vi "Get SMO Public API.vi"(8 "error in (no error)":errorcluster, 11 "Example Instrument in":refnum<class "Instrument.Element2.lvclass">) -> (0 "error out":errorcluster, 2 "Commands":string[](array[string]), 3 "Example Instrument out":refnum<class "Instrument.Element2.lvclass">)   [LabVIEW 2019, in "Instrument.Element2.lvclass"]
uses:
  Instrument.Element2.lvclass
  Typedefs/Instrument.Element2.Commands--Enum.ctl
  <userlib>/LevyLab/Instrument Framework/Instrument Types/VSource/Instrument.VSource.lvclass
  <userlib>/LevyLab/Instrument Framework/SMOs/Instrument/Instrument.lvclass
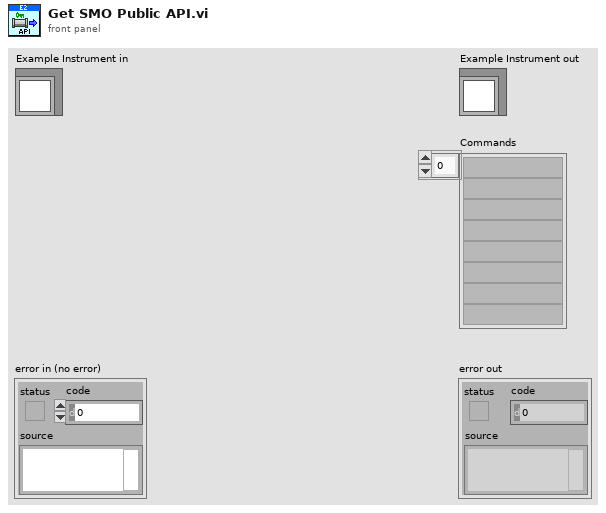
[diagram p1: front panel]
types:
  T1 = typedef "Instrument.Element2.lvclass/Instrument.Element2.Commands--Enum.ctl" = enum16{"command0", "command1", "command2"}
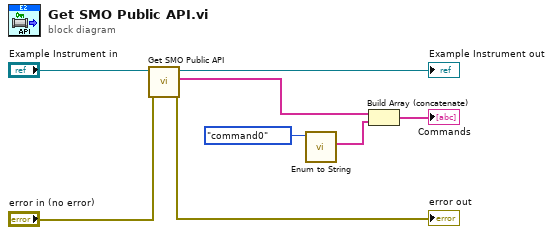
[diagram p0: block diagram]
diagram:
  n1 = call-parent "Get SMO Public API.vi"("error in (no error)"="error in (no error)", "Instrument in"="Example Instrument in") -> ("error out"=→"error out":errorcluster, "Commands"=w8:string[], "Instrument out"=→"Example Instrument out":refnum<class "Instrument.Element2.lvclass">)  [unwired: 7 in]
  n2 = call <userlib>:"Enum to String.vi"("Command"=Instrument.Element2.Commands--Enum."command0" ("Commands")) -> ("Commands []"=w3:string[])  [unwired: 9 in, 1 out]
  n3 = Build Array (concatenate)(w8, w3) -> (→"Commands":string[])
